vi "fgv_timer_e-stop.vi"(7 "cmd":enum16{"check", "start", "pause"}(ring), 8 "error in":errorcluster, 11 "target time":dbl) -> (0 "error out":errorcluster, 2 "time_status_out":T1 {"total time" format="%.1f"; "run time" format="%.1f"; "pause time" format="%.1f"}, 3 "time-out":bool)   [LabVIEW 2019]
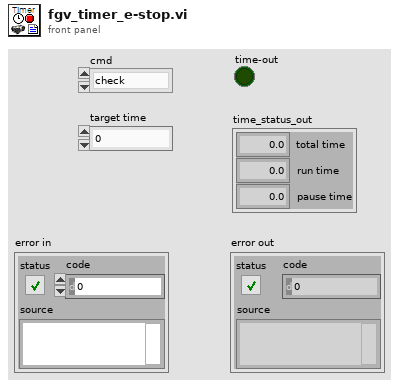
[diagram p1: front panel]
types:
  T1 = cluster{"total time":dbl, "run time":dbl, "pause time":dbl}
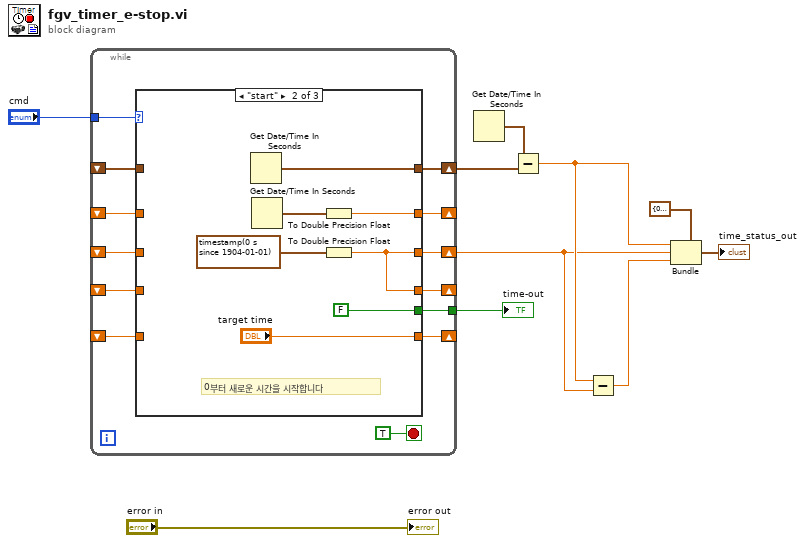
[diagram p0: block diagram]
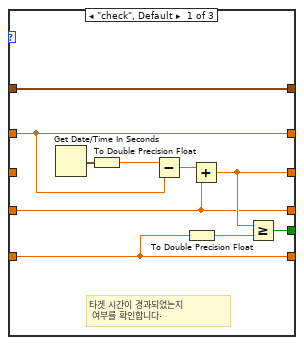
[diagram p2: hidden frame]
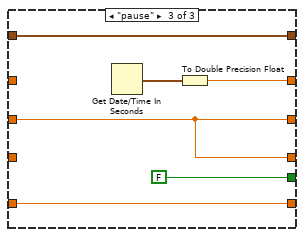
[diagram p3: hidden frame]
diagram:
  n1 = while {
    tunnel: [w22] -> w7
    shift-right: [w21] -> _
    shift-left: _ -> [w20]
    tunnel: "cmd" -> [w19]
    shift-right: [w17] -> w5
    shift-left: _ -> [w18]
    shift-right: [w16] -> _
    shift-left: _ -> [w15]
    shift-right: [w14] -> w9
    shift-left: _ -> [w13]
    shift-right: [w12] -> _
    shift-left: _ -> [w11]
    stop <- TRUE stop-if-true
    n2 = case shown="\"start\"" w19 {
      tunnel: [w29 w38 w44] -> w21
      tunnel: w20 -> [w29 _ _]
      tunnel: [w27 w36 w43] -> w17
      tunnel: [w31 FALSE FALSE] -> w22
      tunnel: w18 -> [_ _ w43]
      tunnel: [w26 w36 w43] -> w16
      tunnel: w15 -> [w26 _ _]
      tunnel: [w25 w35 w42] -> w14
      tunnel: w13 -> [w25 _ w42]
      tunnel: [w24 "target time" w41] -> w12
      tunnel: w11 -> [w24 _ w41]
      frame "check", Default {
        # "타겟 시간이 경과되었는지\n 여부를 확인합니다."
        n3 = Get Date/Time In Seconds() -> (seconds since 1Jan1904=w33:timestamp)
        n4 = To Double Precision Float(number=w33) -> (double precision float=w30:dbl)
        n5 = Subtract(x=w30, y=w29) -> (x-y=w28:dbl)
        n6 = To Double Precision Float(number=w24) -> (double precision float=w32:dbl)
        n7 = Add(x=w28, y=w26) -> (x+y=w27:dbl)
        n8 = Greater Or Equal?(x=w27, y=w32) -> (x >= y?=w31:bool)
      }
      frame "start" {
        # "0부터 새로운 시간을 시작합니다"
        n9 = Get Date/Time In Seconds() -> (seconds since 1Jan1904=w35:timestamp)
        n10 = Get Date/Time In Seconds() -> (seconds since 1Jan1904=w40:timestamp)
        n11 = To Double Precision Float(number=w40) -> (double precision float=w38:dbl)
        n12 = To Double Precision Float(number=timestamp(0 s since 1904-01-01)) -> (double precision float=w36:dbl)
      }
      frame "pause" {
        n13 = Get Date/Time In Seconds() -> (seconds since 1Jan1904=w46:timestamp)
        n14 = To Double Precision Float(number=w46) -> (double precision float=w44:dbl)
      }
    }
  }
  "time-out" <- w7
  n15 = Get Date/Time In Seconds() -> (seconds since 1Jan1904=w8:timestamp)
  n16 = Subtract(x=w8, y=w9) -> (x-y=w6:dbl)
  n17 = Subtract(x=w6, y=w5) -> (x-y=w4:dbl)
  n18 = Bundle(cluster=T1 {"total time"=0.0, "run time"=0.0, "pause time"=0.0} ("output cluster"), "total time"=w6, "run time"=w5, "pause time"=w4) -> (→"time_status_out":T1)
  "error out" <- "error in"
